vi "Can't tell timestamp.vi"() -> ()   [LabVIEW 2017]
panel:
  out "*(type *) &x 2":u64
  out "*(type *) &x":u64
  out "double precision float 2":dbl
  out "double precision float":dbl
  out "current time 2":timestamp
  out "current time":timestamp
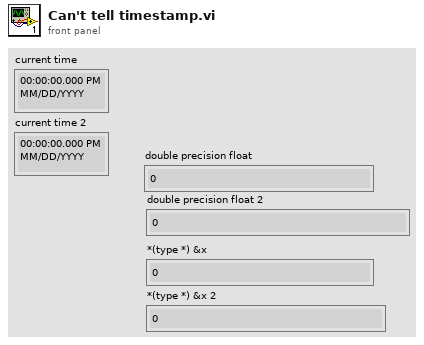
[diagram p1: front panel]
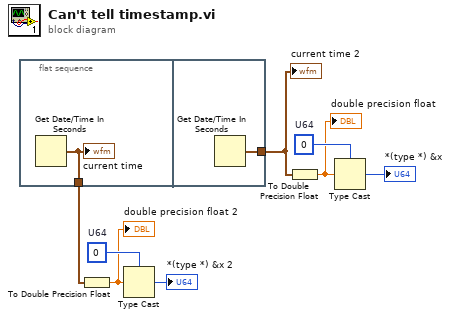
[diagram p0: block diagram]
diagram:
  w7 = u64 0  # U64
  w8 = u64 0  # U64
  n1 = flat-sequence {
    tunnel: [w9] -> w1
    tunnel: [w10] -> w2
    frame #0 {
      n2 = Get Date/Time In Seconds() -> (seconds since 1Jan1904=w9:timestamp)
      "current time" <- w9
    }
    frame #1 {
      n3 = Get Date/Time In Seconds() -> (seconds since 1Jan1904=w10:timestamp)
    }
  }
  n4 = To Double Precision Float(number=w1) -> (double precision float=w6:dbl)
  "double precision float 2" <- w6
  n5 = Type Cast(type=w8, x=w6) -> (*(type *) &x=→"*(type *) &x 2":u64)
  n6 = To Double Precision Float(number=w2) -> (double precision float=w5:dbl)
  "double precision float" <- w5
  n7 = Type Cast(type=w7, x=w5) -> (*(type *) &x=→"*(type *) &x":u64)
  "current time 2" <- w2
